vi "RC_test_2.vi"() -> ()   [LabVIEW 2013]
uses:
  Data/TypeDefs/Rudder Set Suggestions.ctl
  Data/TypeDefs/DynamixelCycleTracker.ctl
  <vilib>/FPGAPlugInAG/myRIO-1900/niLvFpga_Open_myRIO-1900.vi
  <vilib>/rvi/interface/common/dynamic/niFpgaDynamicAddResources.vi
  <vilib>/rvi/interface/nirviOpenFPGA/nirviOpenFPGA.xnode
  FPGA Bitfiles/AutonomousSailbo_FPGATarget_myRIOPWMDecoder_0snwDOwOU4s.lvbitx
  FPGA_Code/myRIO_PWM_Decoder.vi
  <instrlib>/Dynamixel Motor/Dynamixel Motor.lvlib
panel:
  out "Write loop counter":i32
  in  "Read actions per\nwrite action":i32=4
  out "Commanded sail value":dbl
  in  "VISA resource name":refnum<visa-resource-name>="ASRL3::INSTR"
  in  "Stop reading/writing":bool
  out "Read loop counter":i32
  out "Dynamixel\nPositions (deg)":dbl[](array[numeric])
  out "Updated Dynamixel Cycles":T1
  out "error out":errorcluster[](array[cluster])
  in  "Motors Enabled":bool[](array[boolean])=[TRUE, TRUE, TRUE]
  out "Commanded rudder value":T2 min=-0.95 max=0.95 scale=1.0..-1.0
  out "Motors IDs Found":u8[](array[numeric])
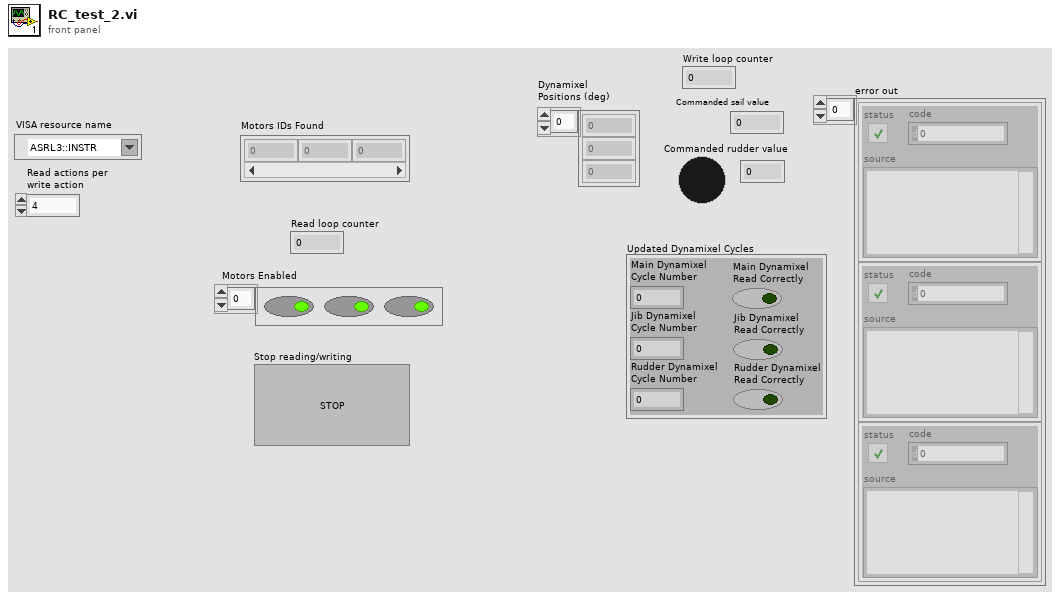
[diagram p1: front panel]
types:
  T1 = typedef "DynamixelCycleTracker.ctl" = cluster{"Main Dynamixel\nCycle Number":i32, "Jib Dynamixel\nCycle Number":i32, "Rudder Dynamixel\nCycle Number":i32, "Main Dynamixel\nRead Correctly":bool, "Jib Dynamixel\nRead Correctly":bool, "Rudder Dynamixel\nRead Correctly":bool}
  T2 = typedef "Rudder Set Suggestions.ctl" = dbl
  T3 = typedef "MotorSetup.ctl" = cluster{"Main Dynamixel Set Data":T4, "Rudder Dynamixel Set Data":T4, "Jib Dynamixel Set Data":T4}
  T4 = typedef "DynamixelSetupInfo.ctl" = cluster{"Lower Winch Bound (deg)":dbl, "Upper Winch Bound (deg)":dbl}
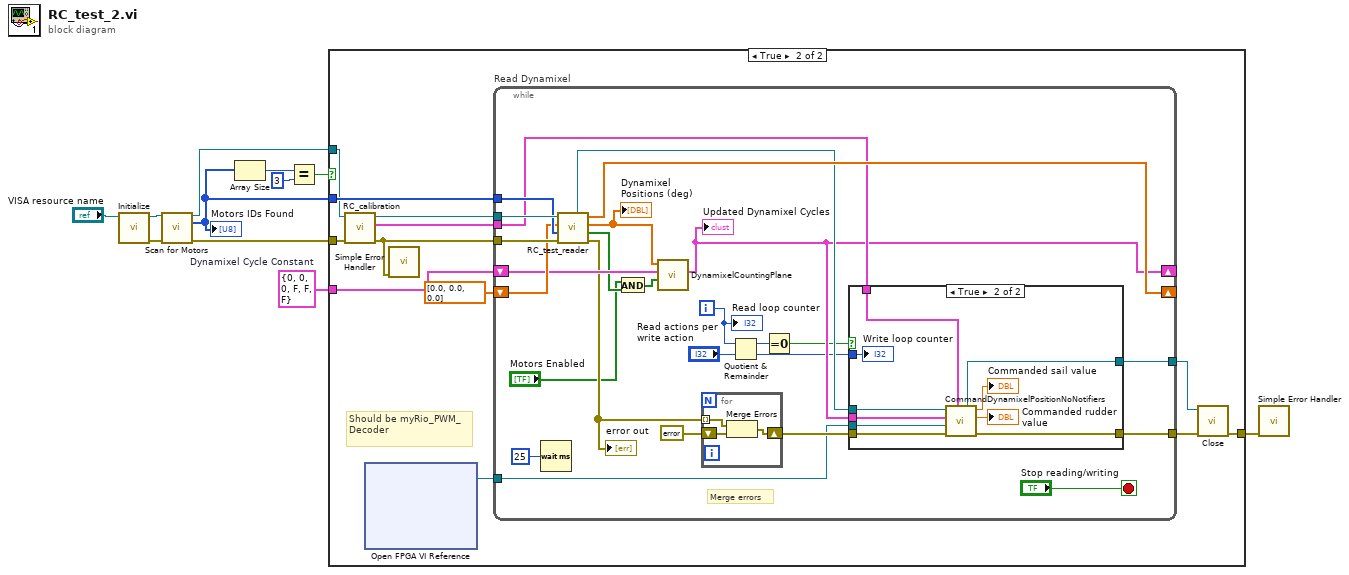
[diagram p0: block diagram]
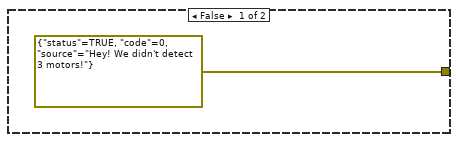
[diagram p2: hidden frame]
diagram:
  w4 = T1 {"Main Dynamixel\nCycle Number"=0, "Jib Dynamixel\nCycle Number"=0, "Rudder Dynamixel\nCycle Number"=0, "Main Dynamixel\nRead Correctly"=FALSE, "Jib Dynamixel\nRead Correctly"=FALSE, "Rudder Dynamixel\nRead Correctly"=FALSE}  # Dynamixel Cycle Constant
  n1 = call <instrlib>:"Initialize.vi"("VISA resource name"="VISA resource name") -> ("error out"=w2:errorcluster, "VISA resource name out"=w3:refnum<visa-resource-name>)  [unwired: 9 in]
  n2 = call <instrlib>:"Scan for Motors.vi"("VISA resource name"=w3, "error in (no error)"=w2) -> ("VISA resource name out"=w5:refnum<visa-resource-name>, "Motors IDs Found"=w11:u8[], "error out"=w6:errorcluster)  [unwired: 11 in]
  "Motors IDs Found" <- w11
  n3 = Array Size(array=w11) -> (size(s)=w7:i32)
  n4 = Equal?(x=w7, y=3) -> (x = y?=w8:bool)
  n5 = case shown="True" w8 {
    tunnel: w4 -> [_ w24]
    tunnel: w11 -> [_ w23]
    tunnel: w5 -> [_ w21]
    tunnel: w6 -> [_ w20]
    tunnel: [errorcluster {"status"=TRUE, "code"=0, "source"="Hey! We didn't detect 3 motors!"} ("error IO") w13] -> w10
    frame False {
    }
    frame True {
      # "Should be myRio_PWM_Decoder"
      n6 = call "RC_calibration.vi"("error in (no error)"=w20, "VISA resource name"=w21) -> ("error IO"=w18:errorcluster, "Dynamixel Bounds Out"=w15:T3, "VISA resource name out"=w19:refnum<visa-resource-name>)  [unwired: 7 in]
      n7 = xnode "Open FPGA VI Reference"() -> ("FPGA VI Reference Out"=w17:refnum<k20>)  [unwired: 2 in, 1 out]
      n8 = call <vilib>:"Simple Error Handler.vi"("error in (no error)"=w18) -> ()  [unwired: 4 in, 5 out]
      n9 = while "Read Dynamixel" {
        tunnel: w19 -> [w49]
        shift-right: [w33] -> _
        shift-left: w24 -> [w42]
        tunnel: w23 -> [w47]
        tunnel: w18 -> [w50]
        shift-right: [w44] -> _
        shift-left: dbl[] [0.0, 0.0, 0.0] -> [w43]
        tunnel: w17 -> [w36]
        tunnel: w15 -> [w35]
        tunnel: [w31] -> w14
        tunnel: [w30] -> w16
        i -> [w29]
        stop <- "Stop reading/writing" stop-if-true
        # "Merge errors"
        n10 = Wait (ms)(milliseconds to wait=u32 25) -> ()  [unwired: 1 out]
        n11 = call "RC_test_reader.vi"("error in (no error)"=w50, "Motors IDs Found"=w47, "Read positions (dyn)"=w43, "VISA Refnum in"=w49) -> ("error out"=w41:errorcluster[], "Motors Read Correctly"=w39:bool[], "Dynamixel Positions (deg)"=w46:dbl[], "Read positions latest (dyn)"=w44:dbl[], "VISA Refnum in 2"=w34:refnum<visa-resource-name>)  [unwired: 3 in]
        "Dynamixel\nPositions (deg)" <- w46
        "error out" <- w41
        n12 = And(x="Motors Enabled", y=w39) -> (x .and. y?=w40:bool[])
        n13 = call "DynamixelCountingPlane.vi"("Motors Read Correctly"=w40, "Dynamixel Cycles"=w42, "Dynamixel Read Positions"=w46) -> ("Updated Dynamixle Cycles"=w33:T1)  [unwired: 8 in]
        "Updated Dynamixel Cycles" <- w33
        n14 = for {
          shift-right: [w65] -> w37
          shift-left: errorcluster {"status"=FALSE, "code"=0, "source"=""} ("error IO") -> [w64]
          tunnel: w41 -> [w63] mode=indexing
          n15 = Merge Errors(w63, w64) -> (w65:errorcluster)
        }
        n16 = Quotient & Remainder(x=w29, y="Read actions per\nwrite action") -> (x-y*floor(x/y)=w27:i32, floor(x/y)=w25:i32)
        n17 = Equal To 0?(x=w27) -> (x = 0?=w26:bool)
        n18 = case shown="True" w26 {
          tunnel: w37 -> [w52 w62]
          tunnel: w36 -> [_ w61]
          tunnel: w35 -> [_ w60]
          tunnel: w34 -> [w51 w59]
          tunnel: w33 -> [_ w58]
          tunnel: [w52 w55] -> w31
          tunnel: [w51 w54] -> w30
          tunnel: w25 -> [_ w53]
          frame False {
          }
          frame True {
            n19 = call "CommandDynamixelPositionNoNotifiers.vi"("Dynamixel Bounds"=w60, "error in"=w62, "FPGA VI Reference In"=w61, "Dynamixel Cycles"=w58, "VISA resource name"=w59) -> ("Error out"=w55:errorcluster, "Commanded rudder value"=→"Commanded rudder value":T2, "Debug sail value"=→"Commanded sail value":dbl, "VISA resource name OUT"=w54:refnum<visa-resource-name>)  [unwired: 3 in]
            "Write loop counter" <- w53
          }
        }
        "Read loop counter" <- w29
      }
      n20 = call <instrlib>:"Close.vi"("error in (no error)"=w14, "VISA resource name"=w16) -> ("error out"=w13:errorcluster)  [unwired: 9 in]
    }
  }
  n21 = call <vilib>:"Simple Error Handler.vi"("error in (no error)"=w10) -> ()  [unwired: 4 in, 5 out]
